vi "joystick_Cov.vi"(11 "Mod State":T1[](array[typedef]) {"Angle"."SIN" format="%13.4f"; "Angle"."COS" format="%13.4f"; "Angle"."VALUE" format="%13.4f"}) -> ()   [LabVIEW 2020]
doc: "takes the joystick input and the gyro angle in radians from global variables and converts them to chassis speeds by multiplying joystick values with the max speed global variable. Then converts chassis speeds to module states. From module states we get module speed(m/s) and angle(r)."
uses:
  <vilib>/Rock Robotics/WPI/ThirdParty/JAS_Junk/TrajLib/TypeDef/SWERVE_DRIVE_MODULE_STATE.ctl
  <vilib>/Rock Robotics/WPI/ThirdParty/JAS_Junk/TrajLib/TypeDef/ROTATION2D.ctl
  <vilib>/Rock Robotics/WPI/Joystick/XBox Buttons Indexer.ctl
  <vilib>/Rock Robotics/WPI/Joystick/XBox Axes Indexer.ctl
  <vilib>/Rock Robotics/WPI/ThirdParty/JAS_Junk/TrajLib/Rotation2d_GetCos.vi
  <vilib>/Rock Robotics/WPI/ThirdParty/JAS_Junk/TrajLib/Rotation2d_GetSin.vi
  <vilib>/Rock Robotics/WPI/ThirdParty/JAS_Junk/TrajLib/ChassisSpeeds_New.vi
  <vilib>/Rock Robotics/WPI/ThirdParty/JAS_Junk/TrajLib/Rotation2d_Minus.vi
  <vilib>/Rock Robotics/WPI/ThirdParty/JAS_Junk/TrajLib/Rotation2d_GetRadians.vi
  <vilib>/Rock Robotics/WPI/ThirdParty/JAS_Junk/TrajLib/SwerveModuleState_New.vi
  <vilib>/Rock Robotics/WPI/ThirdParty/JAS_Junk/TrajLib/Rotation2d_RotateBy.vi
  <vilib>/Rock Robotics/WPI/ThirdParty/JAS_Junk/TrajLib/Rotation2d_UnaryMinus.vi
  <vilib>/Rock Robotics/WPI/ThirdParty/JAS_Junk/TrajLib/Rotation2d_CreateXY.vi
  <vilib>/Rock Robotics/WPI/ThirdParty/JAS_Junk/TrajLib/Util_CalcDist.vi
  Robot Global Data.vi
  <vilib>/Rock Robotics/WPI/ThirdParty/JAS_Junk/TrajLib/Trajectory_Library.lvlib
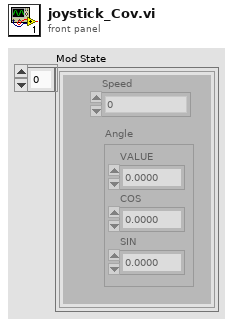
[diagram p1: front panel]
types:
  T1 = typedef "Trajectory_Library.lvlib/SWERVE_DRIVE_MODULE_STATE.ctl" = cluster{"Speed":dbl, "Angle":T2}
  T2 = typedef "Trajectory_Library.lvlib/ROTATION2D.ctl" = cluster{"VALUE":dbl, "COS":dbl, "SIN":dbl}
  T3 = typedef "XBox Buttons Indexer.ctl" = enum16{"A", "B", "X", "Y", "Left Bumper", "Right Bumper", "Back", "Start", "Left Joystick", "Right Joystick"}
  T4 = typedef "XBox Axes Indexer.ctl" = enum16{"Left X", "Left Y", "Left Trigger", "Right Trigger", "Right X", "Right Y"}
  T5 = typedef "Trajectory_Library.lvlib/CHASSIS_SPEEDS.ctl" = cluster{"vX":dbl, "vY":dbl, "vOmega":dbl}
  T6 = typedef "Trajectory_Library.lvlib/SWERVE_DRIVE_KINEMATICS.ctl" = cluster{"NumModules":i32, "InverseKinematics":T7, "ForwardKinematics":T7, "Modules":T8[], "PrevCoR":T8, "SavedModuleStates":T1[]}
  T7 = typedef "NI_Matrix.lvlib/RealMatrix.ctl" = dbl[][]
  T8 = typedef "Trajectory_Library.lvlib/TRANSLATION2D.ctl" = cluster{"X":dbl, "Y":dbl}
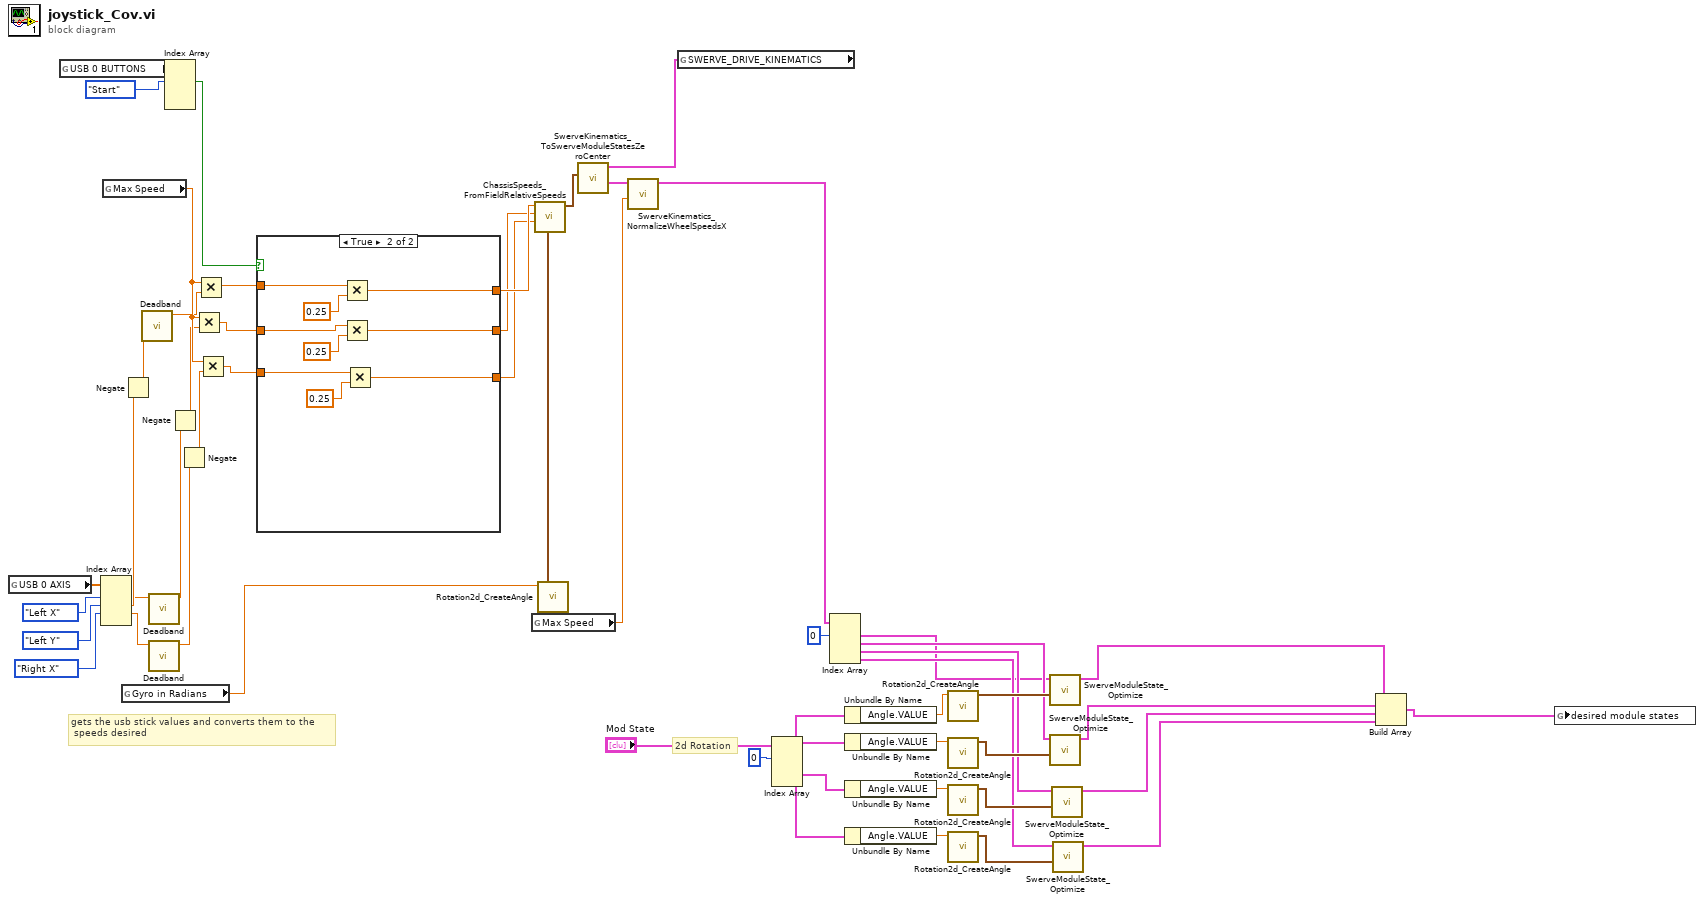
[diagram p0: block diagram]
diagram:
  # "gets the usb stick values and converts them to the\n speeds desired"
  # "2d Rotation"
  n1 = global read "Robot Global Data.vi" "USB 0 AXIS"() -> (w46:dbl[])
  n2 = global read "Robot Global Data.vi" "USB 0 BUTTONS"() -> (w9:bool[])
  n3 = Index Array(array=w46, index #1=XBox_Axes_Indexer."Left X" ("XBox Axes"), index #2=XBox_Axes_Indexer."Left Y" ("XBox Axes"), index #3=XBox_Axes_Indexer."Right X" ("XBox Axes")) -> (element #1=w40:dbl, element #2=w41:dbl, element #3=w42:dbl)  [unwired: 1 in, 1 out]
  n4 = global read "Robot Global Data.vi" "Max Speed"() -> (w50:dbl)
  n5 = global read "Robot Global Data.vi" "Gyro in Radians"() -> (w51:dbl)
  n6 = Negate(x=w41) -> (-x=w3:dbl)
  n7 = call "Deadband.vi"("upper limit"=w3) -> ("Numeric"=w38:dbl)  [unwired: 9 in, 1 out]
  n8 = call "Deadband.vi"("upper limit"=w40) -> ("Numeric"=w39:dbl)  [unwired: 9 in, 1 out]
  n9 = call "Deadband.vi"("upper limit"=w42) -> ("Numeric"=w37:dbl)  [unwired: 9 in, 1 out]
  n10 = Index Array(array=w9, index #1=XBox_Buttons_Indexer."Start" ("XBox Buttons")) -> (element #1=w7:bool)  [unwired: 3 in, 3 out]
  n11 = Negate(x=w39) -> (-x=w2:dbl)
  n12 = Negate(x=w37) -> (-x=w1:dbl)
  n13 = Multiply(x=w50, y=w2) -> (x*y=w6:dbl)
  n14 = Multiply(x=w50, y=w38) -> (x*y=w12:dbl)
  n15 = Multiply(x=w50, y=w1) -> (x*y=w13:dbl)
  n16 = case shown="True" w7 {
    tunnel: w13 -> [w56 w65]
    tunnel: w12 -> [w57 w62]
    tunnel: [w57 w61] -> w11
    tunnel: [w55 w60] -> w5
    tunnel: [w56 w59] -> w10
    tunnel: w6 -> [w55 w58]
    frame False {
    }
    frame True {
      n17 = Multiply(x=w62, y=0.25) -> (x*y=w61:dbl)
      n18 = Multiply(x=w58, y=0.25) -> (x*y=w60:dbl)
      n19 = Multiply(x=w65, y=0.25) -> (x*y=w59:dbl)
    }
  }
  n20 = global read "Robot Global Data.vi" "Max Speed"() -> (w17:dbl)
  n21 = call <vilib>:"Rotation2d_CreateAngle.vi"("Angle"=w51) -> ("ROTATION"=w52:T2)  [unwired: 10 in]
  n22 = call <vilib>:"ChassisSpeeds_FromFieldRelativeSpeeds.vi"("RobotAngle"=w52, "Omega"=w10, "vY"=w5, "vX"=w11) -> ("CHASSIS"=w53:T5)  [unwired: 7 in]
  n23 = global read "Robot Global Data.vi" "SWERVE_DRIVE_KINEMATICS"() -> (w54:T6)
  n24 = call <vilib>:"SwerveKinematics_ToSwerveModuleStatesZeroCenter.vi"("ChassisSpeeds"=w53, "in SWERVE_DRIVE_KINEMATICS"=w54) -> ("ModuleStates"=w44:T1[])  [unwired: 8 in, 1 out]
  n25 = call <vilib>:"SwerveKinematics_NormalizeWheelSpeedsX.vi"("AttainableMaxSpeed"=w17, "in WheelStates"=w44) -> ("out WheelStates"=w43:T1[])  [unwired: 9 in]
  n26 = Index Array(array="Mod State", index #1=0 ("index")) -> (element #1=w14:T1, element #2=w30:T1, element #3=w29:T1, element #4=w28:T1)  [unwired: 3 in]
  n27 = Index Array(array=w43, index #1=0 ("index")) -> (element #1=w15:T1, element #2=w23:T1, element #3=w22:T1, element #4=w21:T1)  [unwired: 3 in]
  n28 = Unbundle By Name(w14) -> ("Angle.VALUE"=w34:dbl)
  n29 = Unbundle By Name(w30) -> ("Angle.VALUE"=w33:dbl)
  n30 = Unbundle By Name(w29) -> ("Angle.VALUE"=w32:dbl)
  n31 = Unbundle By Name(w28) -> ("Angle.VALUE"=w31:dbl)
  n32 = call <vilib>:"Rotation2d_CreateAngle.vi"("Angle"=w34) -> ("ROTATION"=w27:T2)  [unwired: 10 in]
  n33 = call <vilib>:"Rotation2d_CreateAngle.vi"("Angle"=w33) -> ("ROTATION"=w26:T2)  [unwired: 10 in]
  n34 = call <vilib>:"Rotation2d_CreateAngle.vi"("Angle"=w32) -> ("ROTATION"=w25:T2)  [unwired: 10 in]
  n35 = call <vilib>:"Rotation2d_CreateAngle.vi"("Angle"=w31) -> ("ROTATION"=w24:T2)  [unwired: 10 in]
  n36 = call <vilib>:"SwerveModuleState_Optimize.vi"("CurrentAngle"=w27, "Desired State"=w15) -> ("out SWERVE_DRIVE_MODULE_STATE"=w16:T1)  [unwired: 9 in]
  n37 = call <vilib>:"SwerveModuleState_Optimize.vi"("CurrentAngle"=w26, "Desired State"=w23) -> ("out SWERVE_DRIVE_MODULE_STATE"=w20:T1)  [unwired: 9 in]
  n38 = call <vilib>:"SwerveModuleState_Optimize.vi"("CurrentAngle"=w25, "Desired State"=w22) -> ("out SWERVE_DRIVE_MODULE_STATE"=w19:T1)  [unwired: 9 in]
  n39 = call <vilib>:"SwerveModuleState_Optimize.vi"("CurrentAngle"=w24, "Desired State"=w21) -> ("out SWERVE_DRIVE_MODULE_STATE"=w18:T1)  [unwired: 9 in]
  n40 = Build Array(w16, w20, w19, w18) -> (w4:T1[])
  n41 = global write "Robot Global Data.vi" "desired module states"(w4) -> ()
